vi "Set Light.vi"(6 "State":T1, 7 "Light Select":T2, 8 "error in":errorcluster, 11 "Light Stack in":refnum<class "Light Stack.lvclass">) -> (0 "error out":errorcluster, 3 "Light Stack out":refnum<class "Light Stack.lvclass">)   [LabVIEW 2018, in "Light Stack.lvlib" / "Light Stack.lvclass"]
uses:
  Light Stack.lvclass
  Custom Controls/Light Select.ctl
  Custom Controls/Light Mode.ctl
  Light Stack.lvclass/Light Stack.ctl
  Light Stack.lvlib
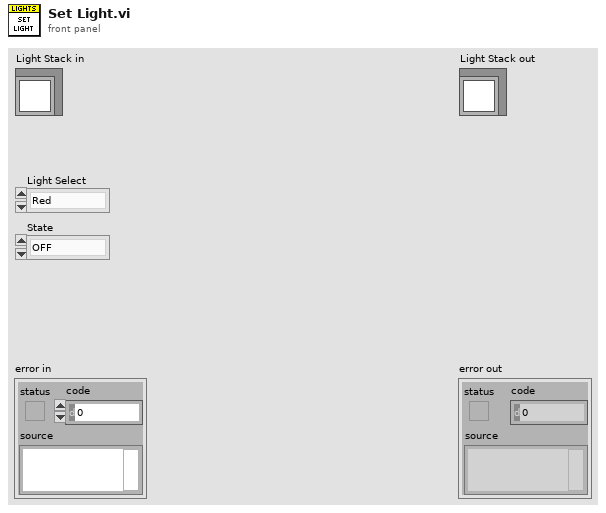
[diagram p1: front panel]
types:
  T1 = typedef "Light Stack.lvlib/Light Mode.ctl" = enum16{"OFF", "ON", "BLINK"}
  T2 = typedef "Light Stack.lvlib/Light Select.ctl" = enum16{"Red", "Amber", "Green", "Blue"}
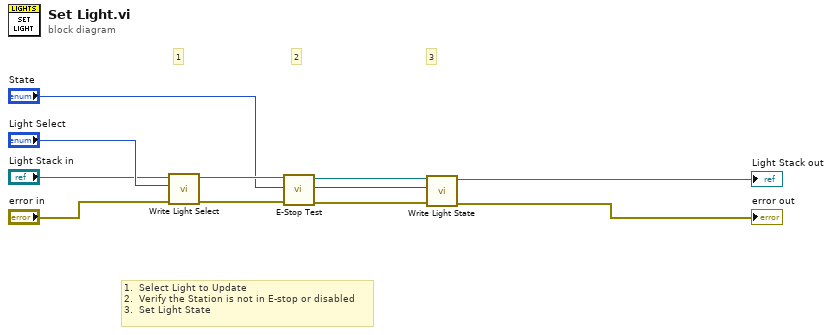
[diagram p0: block diagram]
diagram:
  # "1.  Select Light to Update\n2.  Verify the Station is not in E-stop or disabled\n3.  Set Light State"
  # "3"
  # "2"
  # "1"
  n1 = call "Write Light Select.vi"("error in (no error)"="error in", "Light Select"="Light Select", "Light Stack in"="Light Stack in") -> ("error out"=w8:errorcluster, "Light Stack out"=w7:refnum<class "Light Stack.lvclass">)  [unwired: 7 in]
  n2 = call "E-Stop Test.vi"("error in"=w8, "State"="State", "Light Stack in"=w7) -> ("error out"=w3:errorcluster, "Output State"=w5:T1, "Light Stack out"=w4:refnum<class "Light Stack.lvclass">)  [unwired: 6 in]
  n3 = call "Write Light State.vi"("error in"=w3, "Light Mode"=w5, "Light Stack in"=w4) -> ("error out"=→"error out":errorcluster, "Light Stack out"=→"Light Stack out":refnum<class "Light Stack.lvclass">)  [unwired: 7 in]
